vi "Read Box.vi"(0 "Wait (ms)":u32=50, 1 "Timeout (ms)":i32=1000, 2 "# Tries":i32=4, 3 "GPIB Address":string="15", 4 "# Iterations":i32=2) -> (6 "Error Reading":errorcluster, 7 "Reading":string[](array[string]), 9 "Error Writing":errorcluster)   [LabVIEW 2009]
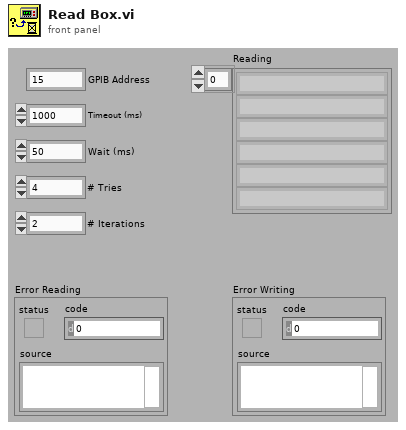
[diagram p1: front panel]
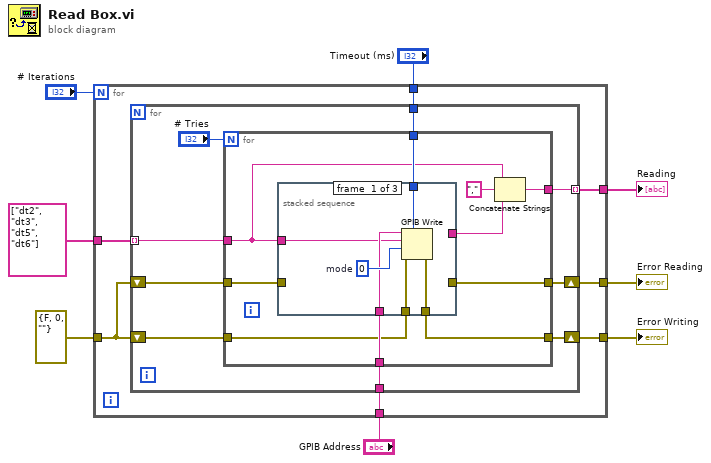
[diagram p0: block diagram]
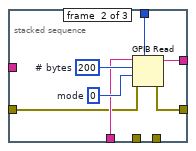
[diagram p2: hidden frame]
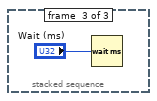
[diagram p3: hidden frame]
diagram:
  n1 = for {
    N: "# Iterations" -> [_]
    tunnel: [w15] -> w8
    tunnel: [w14] -> w7
    tunnel: "GPIB Address" -> [w13]
    tunnel: "Timeout (ms)" -> [w12]
    tunnel: errorcluster {"status"=FALSE, "code"=0, "source"=""} ("error out") -> [w9]
    tunnel: [w11] -> w1
    tunnel: string[] ["dt2", "dt3", "dt5", "dt6"] -> [w10]
    n2 = for {
      tunnel: w13 -> [w22]
      tunnel: w12 -> [w21]
      tunnel: [w20] -> w11 mode=indexing
      tunnel: w10 -> [w19] mode=indexing
      shift-right: [w24] -> w15
      shift-left: w9 -> [w17]
      shift-right: [w23] -> w14
      shift-left: w9 -> [w16]
      n3 = for {
        N: "# Tries" -> [_]
        tunnel: [w34] -> w20
        tunnel: w22 -> [w33]
        tunnel: w21 -> [w29]
        tunnel: w19 -> [w25]
        tunnel: w17 -> [w27]
        tunnel: [w32] -> w24
        tunnel: w16 -> [w26]
        tunnel: [w31] -> w23
        n4 = stacked-sequence {
          tunnel: w33 -> [w37 w45 _]
          tunnel: [_ w44 _] -> w32
          tunnel: [w40 _ _] -> w31
          tunnel: [_ w43 _] -> w28
          tunnel: w29 -> [w39 w42 _]
          tunnel: w25 -> [w36 _ _]
          tunnel: w27 -> [_ w41 _]
          tunnel: w26 -> [w35 _ _]
          frame #0 {
            w38 = i16 0  # mode
            n5 = GPIB Write(0:w37, 1:w36, 2:w38, 3:w35, 4:w39) -> (6:w40:errorcluster)  [unwired: 1 out]
          }
          frame #1 {
            w46 = i16 0  # mode
            w47 = 200  # # bytes
            n6 = GPIB Read(0:w45, 1:w47, 2:w46, 3:w41, 4:w42) -> (5:w43:string, 7:w44:errorcluster)  [unwired: 1 out]
          }
          frame #2 {
            n7 = Wait (ms)(milliseconds to wait="Wait (ms)") -> ()  [unwired: 1 out]
          }
        }
        n8 = Concatenate Strings(w25, "," ("string"), w28) -> (w34:string)
      }
    }
  }
  "Reading" <- w1
  "Error Reading" <- w8
  "Error Writing" <- w7
